vi "AREA OF TRIANGLE.vi"() -> ()   [LabVIEW 2022 SP3]
panel:
  out "Area of Triangle":dbl
  out "Validity of triangles":bool
  in  "Side C":dbl=10.0
  in  "Side B":dbl=8.0
  in  "Side A":dbl=6.0
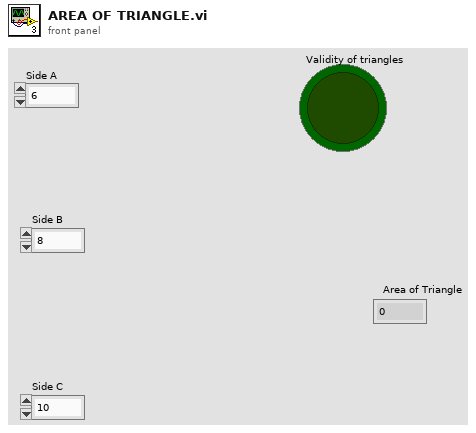
[diagram p1: front panel]
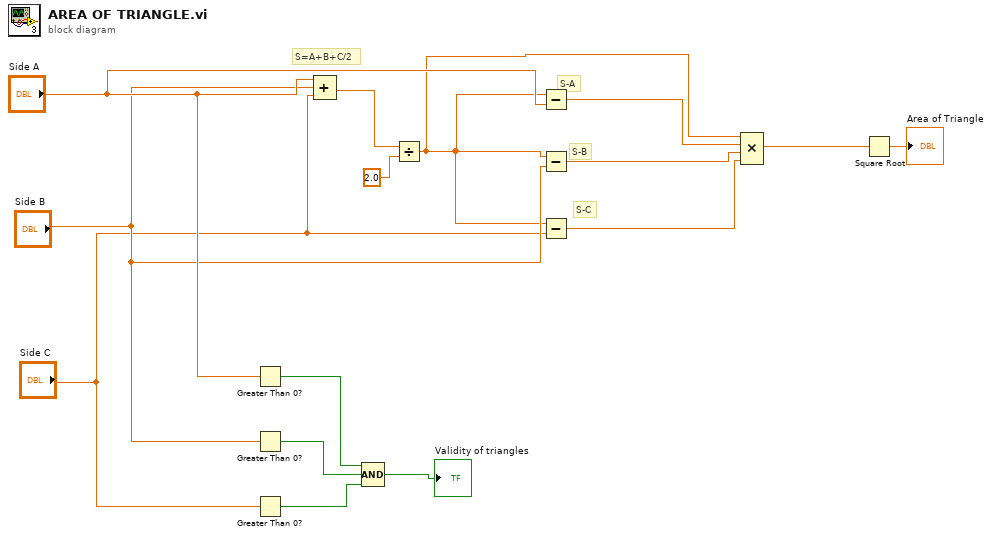
[diagram p0: block diagram]
diagram:
  # "S-C"
  # "S-B"
  # "S-A"
  # "S=A+B+C/2"
  n1 = Greater Than 0?(x="Side A") -> (x > 0?=w13:bool)
  n2 = Greater Than 0?(x="Side B") -> (x > 0?=w14:bool)
  n3 = Greater Than 0?(x="Side C") -> (x > 0?=w15:bool)
  n4 = Compound Arithmetic op=ADD("Side A", "Side B", "Side C") -> (w11:dbl)
  n5 = Compound Arithmetic op=AND(w13, w14, w15) -> (→"Validity of triangles":bool)
  n6 = Divide(x=w11, y=2.0) -> (x/y=w6:dbl)
  n7 = Subtract(x=w6, y="Side A") -> (x-y=w5:dbl)
  n8 = Subtract(x=w6, y="Side B") -> (x-y=w3:dbl)
  n9 = Subtract(x=w6, y="Side C") -> (x-y=w4:dbl)
  n10 = Compound Arithmetic op=MULTIPLY(w6, w5, w3, w4) -> (w2:dbl)
  n11 = Square Root(x=w2) -> (sqrt(x)=→"Area of Triangle":dbl)
